vi "Draw South Wall.vi"(4 "pen":T1={"Width"=2, "Style"=enum."Solid"}, 6 "color":u32(colorbox)=11841024, 7 "Grid Size (10)":i32=10, 8 "Connected":bool, 9 "Col":i32, 10 "Row":i32, 11 "Picture In":picture) -> (3 "Picture":picture)   [LabVIEW 2020, in "App.lvlib" / "MazeUI.lvclass"]
uses:
  MazeUI.lvclass
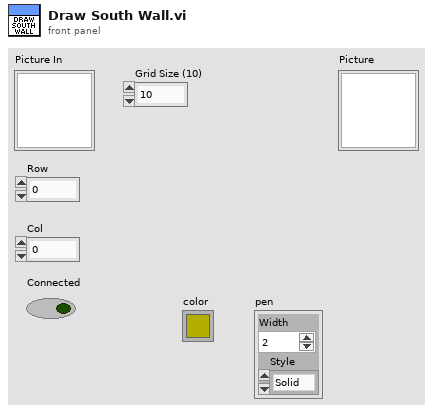
[diagram p1: front panel]
types:
  T1 = cluster{"Width":u16, "Style":enum32{"Solid", "Dash", "Dot", "DashDot", "DashDotDot"}}
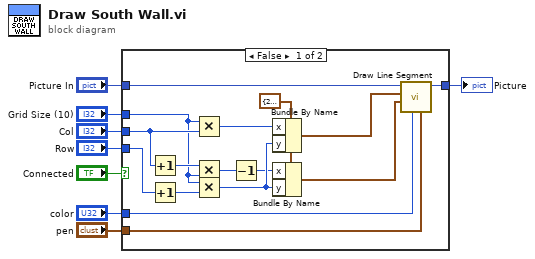
[diagram p0: block diagram]
diagram:
  n1 = case shown="False" "Connected" {
    tunnel: "Picture In" -> [w22 w25]
    tunnel: "Grid Size (10)" -> [w12 _]
    tunnel: "Row" -> [w24 _]
    tunnel: "Col" -> [w15 _]
    tunnel: "color" -> [w18 _]
    tunnel: "pen" -> [w17 _]
    tunnel: [w16 w25] -> w1
    frame False {
      w20 = cluster{"x":i16, "y":i16} {"x"=20, "y"=10} ("Start")
      n2 = Increment(x=w15) -> (x+1=w13:i32)
      n3 = Increment(x=w24) -> (x+1=w23:i32)
      n4 = Multiply(x=w12, y=w15) -> (x*y=w11:i32)
      n5 = Multiply(x=w13, y=w12) -> (x*y=w14:i32)
      n6 = Multiply(x=w12, y=w23) -> (x*y=w10:i32)
      n7 = Decrement(x=w14) -> (x-1=w9:i32)
      n8 = Bundle By Name(cluster=w20, "x"=w11, "y"=w10) -> (w21:cluster{"x":i16, "y":i16})
      n9 = Bundle By Name(cluster=w20, "x"=w9, "y"=w10) -> (w19:cluster{"x":i16, "y":i16})
      n10 = call "Draw Line Segment.vi"("pen"=w17, "color"=w18, "End"=w19, "Start"=w21, "Picture In (New)"=w22) -> ("Picture"=w16:picture)  [unwired: 6 in]
    }
    frame True {
    }
  }
  "Picture" <- w1
